vi "SpecGlbs.vi"() -> ()   [LabVIEW 2011]
panel:
  in  "DisabledTmpSfty":bool
  in  "Single Zone":bool
  in  "Post Warning":bool
  in  "Current Ind":i32[](array[numeric])
  in  "Abort Run":bool
  in  "Channel Ind":i16[][](array[numeric])
  in  "Response Seq":T1(array[ring])=[enum."Warning/Abort"]
  in  "High Limits":dbl[](array[numeric])=[950.0] format="%.2f"
  in  "High Bands":dbl[](array[numeric])=[100.0] format="%.2f"
  in  "Low Bands":dbl[](array[numeric])=[75.0] format="%.2f"
  in  "SpiltScl Chs":i16[](array[numeric])
  in  "Bath Temp":T2={"Bath Port#"=3, "Spare1"=0, "Spare2"=0, "Spare3"=0, "IO Chs"=[]}
  in  "Motor Port#":u16
  in  "Tweek Disable":bool
  in  "GaNzilla Bobcat System":bool
  in  "TGV Set_Driver":sgl=100.0 format="%.2f"
  in  "TGA N2_Time":u32=90
  in  "GC_Exh":i16
  in  "Alcatel":T3={"Alk_Vac"=26, "Covectron"=55, "Manul"="W"}
  in  "Thru_Val":i16=123
  in  "Spindle":cluster{"Fault":i32, "Enable":i32}
  in  "PyriteCtrl":cluster{"Pyrites":i32[], "Din":i32}
  in  "Ion Delay":u32=10000
  in  "Chk GV Press":T4={"Ion Gauge"=70, "Convectron"=71, "I/G"=170, "D/G"=171, "Pressure"=1.0} {"Pressure" format="%.2e"}
  in  "AnteChamber":T5 {"MFC"."Purge Flow" format="%.2f"; "Switch Pressure" format="%.2f"}
  in  "Ion Lock":dbl=0.023 format="%.3f"
  in  "Spec_PD":T6={"PD_cells"=[], "PD Msg"=["", "", ""]}
  in  "Molec Pump":cluster{"Pump+(ms)":u32, "Pump-(ms)":u32}={"Pump+(ms)"=20000, "Pump-(ms)"=15000}
  in  "Spare":cluster{"SpareD":bool[], "SpareA":bool[]}
  # "Temp Safety"
  # "ServoMotor Ctrl"
  # "Motor Control"
  # "NOTES:\n-For systems without direct drive Empty the\n Spindle cluster.\n-For Ganzilla Bobcats selct the GaNzilla Bobcat\n system. This will keep the motor drive enabled in\n all system states.\n-For some systems that do not have std motor\n control (5916), please enable this option."
  # "NOTES:\nThis Feature is used with the \nsystems that have dual exhaust\nvalves for the GC. Leave it = 0 \nfor ALL other systems."
  # "NOTES:\n-Used for P75 systems"
  # "Value is 0 based"
  # "Value is 1 based"
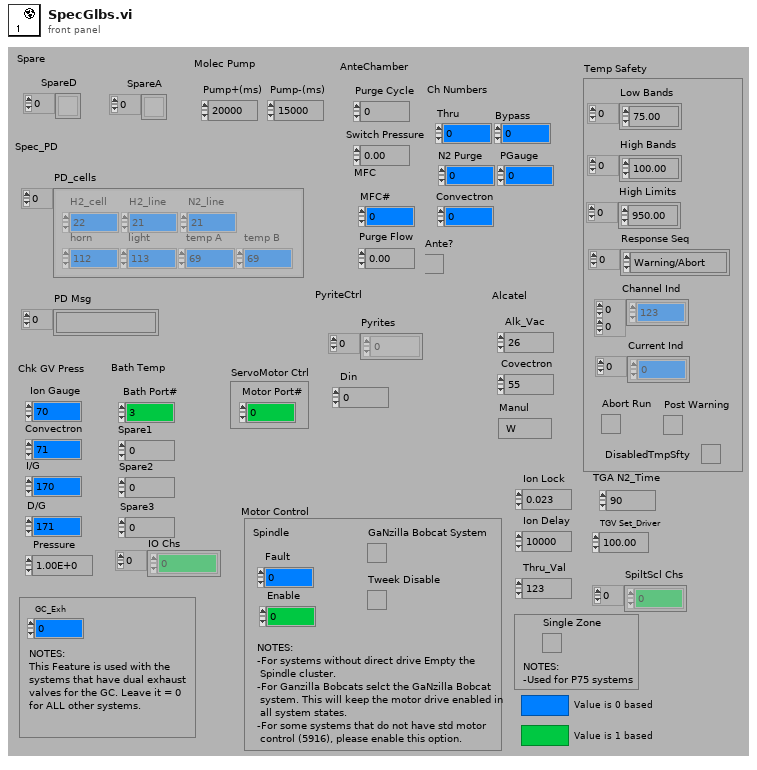
[diagram p1: front panel]
types:
  T1 = enum16{"No Action", "Warning/Abort", "Warning", "Abort", "Shutdown", "Delayed Abort"}[]
  T2 = cluster{"Bath Port#":u16, "Spare1":u16, "Spare2":u16, "Spare3":u16, "IO Chs":u16[]}
  T3 = cluster{"Alk_Vac":i32, "Covectron":i32, "Manul":string}
  T4 = cluster{"Ion Gauge":i32, "Convectron":i32, "I/G":i32, "D/G":i32, "Pressure":dbl}
  T5 = cluster{"Purge Cycle":u8, "Switch Pressure":dbl, "Ch Numbers":cluster{"Thru ":i32, "Bypass":i32, "N2 Purge":i32, "PGauge":i32, "Convectron":i32}, "Ante?":bool, "MFC":cluster{"MFC#":i32, "Purge Flow":dbl}}
  T6 = cluster{"PD_cells":cluster{"H2_cell":u8, "H2_line":u8, "N2_line":u8, "horn":u8, "light":u8, "temp A":u8, "temp B":u8}[], "PD Msg":string[]}
diagram:
